vi "stopGetClientStatus.vi"(8 "error in (no error)":errorcluster, 11 "tcpServer in":refnum<class "TcpServer.lvclass">) -> (0 "error out":errorcluster, 3 "tcpServer out":refnum<class "TcpServer.lvclass">)   [LabVIEW 2018, in "TcpServer.lvclass"]
doc: "Stop the getClientStatus.vi."
uses:
  TcpServer.lvclass
  TcpServer.lvclass/TcpServer.ctl
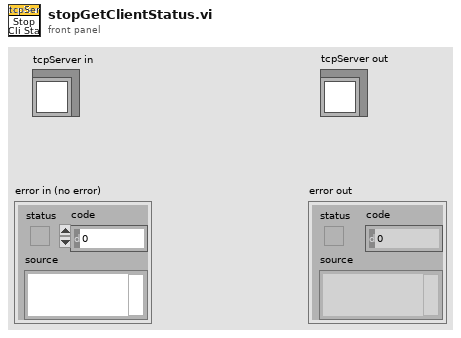
[diagram p1: front panel]
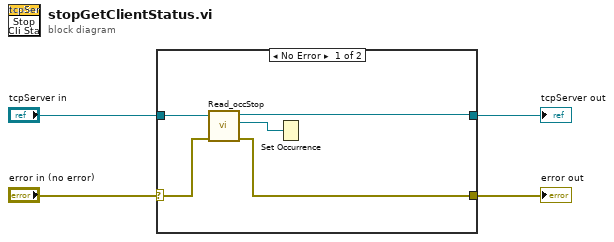
[diagram p0: block diagram]
diagram:
  n1 = case shown="No Error" "error in (no error)" {
    selector: "error in (no error)" -> [w8 w11]
    tunnel: [w5 w11] -> w3
    tunnel: "tcpServer in" -> [w9 w10]
    tunnel: [w6 w10] -> w1
    frame No Error {
      n2 = call "Read_occStop.vi"("error in (no error)"=w8, "TcpServer in"=w9) -> ("error out"=w5:errorcluster, "occStop"=w7:refnum<k4>, "TcpServer out"=w6:refnum<class "TcpServer.lvclass">)  [unwired: 7 in]
      n3 = Set Occurrence(w7) -> ()
    }
    frame Error {
    }
  }
  "error out" <- w3
  "tcpServer out" <- w1
